vi "Utility Write To Register - Floating Point.vi"(0 "VISA resource name":refnum<visa-resource-name>, 1 "Unit Address (1)":u8=1, 5 "Register Address (0)":u16, 9 "Data (0)":sgl format="%.3f", 11 "error in (no error)":errorcluster) -> (4 "VISA resource name out":refnum<visa-resource-name>, 15 "error out":errorcluster)   [LabVIEW 2010, in "Eurotherm 32xx Series.lvlib"]
doc: "This VI writes the values to the specified registers of specified unit."
uses:
  <instrlib>/Eurotherm 32xx Series/Eurotherm 32xx Series.lvlib
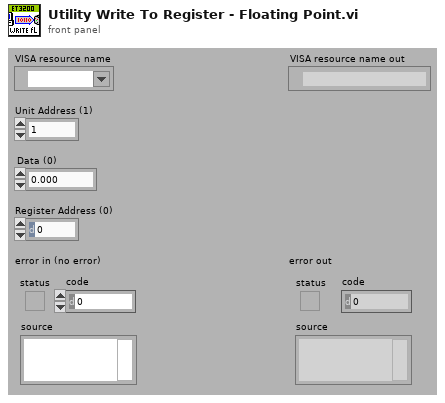
[diagram p1: front panel]
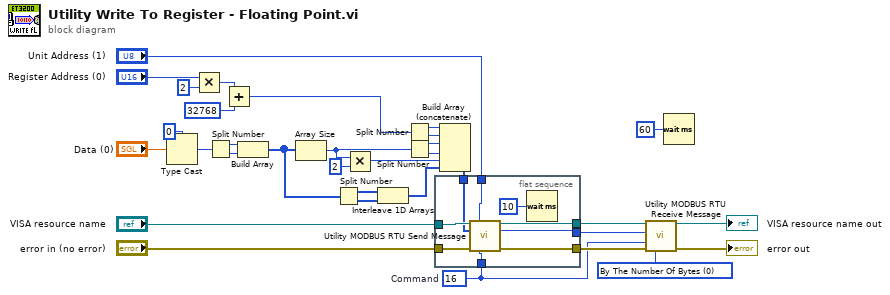
[diagram p0: block diagram]
diagram:
  w1 = u16 0 items=["By The Number Of Bytes", "Copy Of The Sent Message"] ("Receive Message Type (0: By The Number Of Bytes)")
  w28 = u8 16  # Command
  n1 = Type Cast(type=0 ("y"), x="Data (0)") -> (*(type *) &x=w13:i32)
  n2 = Multiply(x="Register Address (0)", y=u16 2) -> (x*y=w8:u16)
  n3 = Split Number(x=w13) -> (hi(x)=w4:u16, lo(x)=w3:u16)
  n4 = Add(x=w8, y=u16 32768) -> (x+y=w5:u16)
  n5 = Build Array(w4, w3) -> (w10:u16[])
  n6 = Array Size(array=w10) -> (size(s)=w19:i32)
  n7 = Split Number(x=w10) -> (hi(x)=w15:u8[], lo(x)=w16:u8[])
  n8 = Multiply(x=w19, y=2) -> (x*y=w18:i32)
  n9 = Interleave 1D Arrays(w15, w16) -> (w14:u8[])
  n10 = Split Number(x=w5) -> (hi(x)=w26:u8, lo(x)=w25:u8)
  n11 = Split Number(x=w19) -> (hi(x)=w24:u16, lo(x)=w23:u16)
  n12 = flat-sequence {
    tunnel: "VISA resource name" -> [w42]
    tunnel: "error in (no error)" -> [w41]
    tunnel: [w40] -> w30
    tunnel: [w39] -> w29
    tunnel: w28 -> [w38]
    tunnel: w27 -> [w37]
    tunnel: [w36] -> w22
    tunnel: "Unit Address (1)" -> [w35]
    frame #0 {
      n13 = call <instrlib>:"Utility MODBUS RTU Send Message.vi"("VISA resource name"=w42, "Unit Address (1)"=w35, "Message (empty array)"=w37, "error in (no error)"=w41, "Command (0)"=w38) -> ("VISA resource name out"=w39:refnum<visa-resource-name>, "Length Of Sent MSG"=w36:u8, "error out"=w40:errorcluster)  [unwired: 8 in]
      n14 = Wait (ms)(milliseconds to wait=u32 10) -> ()  [unwired: 1 out]
    }
  }
  n15 = Build Array (concatenate)(w26, w25, w24, w23, w18, w14) -> (w27:i32[])
  n16 = call <instrlib>:"Utility MODBUS RTU Receive Message.vi"("VISA resource name"=w29, "Length Of Sent MSG (0)"=w22, "Sent Command (0)"=w28, "error in (no error)"=w30, "Receive Message Type (0: By The Number Of Bytes)"=w1) -> ("VISA resource name out"=→"VISA resource name out":refnum<visa-resource-name>, "error out"=→"error out":errorcluster)  [unwired: 8 in, 1 out]
  n17 = Wait (ms)(milliseconds to wait=u32 60) -> ()  [unwired: 1 out]
